vi "test.vi"() -> ()   [LabVIEW 2021]
uses:
  Moving_Statistic.lvclass
panel:
  in  "milliseconds to wait":u32=1000
  out "output cluster":T1
  in  "stop":bool
  in  "Window":i32
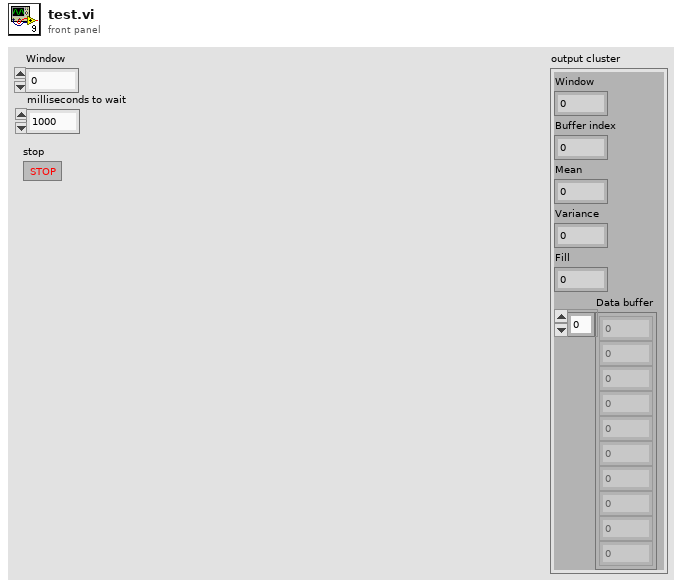
[diagram p1: front panel]
types:
  T1 = cluster{"Window":i32, "Buffer index":i32, "Mean":dbl, "Variance":dbl, "Fill":i32, "Data buffer":dbl[]}
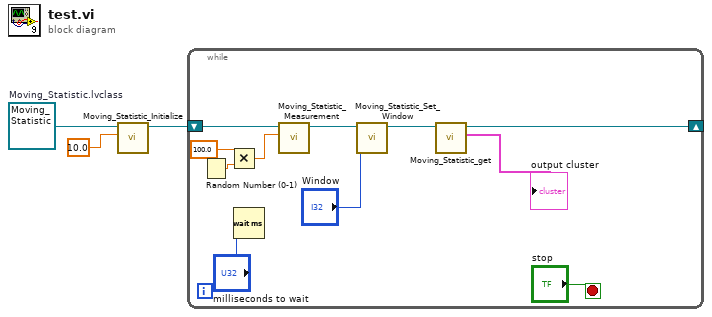
[diagram p0: block diagram]
diagram:
  w3 = refnum<class "Moving_Statistic.lvclass"> refnum  # Moving_Statistic.lvclass
  n1 = call-dynamic "Moving_Statistic_Initialize.vi"("Window"=10.0, "Moving_Mean in"=w3) -> ("Moving_Mean out"=w2:refnum<class "Moving_Statistic.lvclass">)  [unwired: 8 in, 1 out]
  n2 = while {
    shift-right: [w10] -> _
    shift-left: w2 -> [w13]
    stop <- "stop" stop-if-true
    n3 = Random Number (0-1)() -> (number: 0 to 1=w8:dbl)
    n4 = Multiply(x=100.0, y=w8) -> (x*y=w6:dbl)
    n5 = Wait (ms)(milliseconds to wait="milliseconds to wait") -> ()  [unwired: 1 out]
    n6 = call-dynamic "Moving_Statistic_Measurement.vi"("New_Measurement"=w6, "Moving_Mean in"=w13) -> ("Moving_Mean out"=w12:refnum<class "Moving_Statistic.lvclass">)  [unwired: 8 in, 1 out]
    n7 = call-dynamic "Moving_Statistic_Set_Window.vi"("Window"="Window", "Moving_Statistic in"=w12) -> ("Moving_Statistic out"=w11:refnum<class "Moving_Statistic.lvclass">)  [unwired: 8 in, 1 out]
    n8 = call-dynamic "Moving_Statistic_get.vi"("Moving_Statistic in"=w11) -> ("output cluster"=→"output cluster":T1, "Moving_Statistic out"=w10:refnum<class "Moving_Statistic.lvclass">)  [unwired: 8 in, 1 out]
  }
